vi "TDMS File Initialization (Poly).vi"   [LabVIEW 2020]
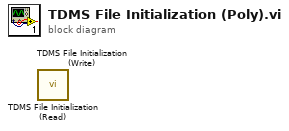
[diagram p0: block diagram]
diagram:
  n1 = call "TDMS File Initialization (Read).vi"() -> ()  [unwired: 8 in, 4 out]
  n2 = call "TDMS File Initialization (Write).vi"() -> ()  [unwired: 8 in, 4 out]
